vi "ForcedJump.vi"(8 "Current Index":dbl, 11 "Offset":dbl) -> (3 "New Index":dbl)   [LabVIEW 2013]
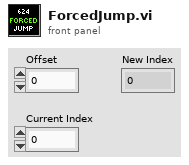
[diagram p1: front panel]
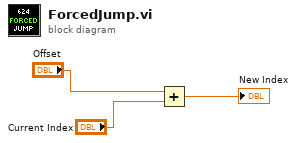
[diagram p0: block diagram]
diagram:
  n1 = Add(x="Offset", y="Current Index") -> (x+y=→"New Index":dbl)
